vi "Initialise Indegrees1.vi"(8 "error in (no error)":errorcluster, 11 "Topological Sort in":refnum<class "Topological Sort.lvclass">) -> (0 "error out":errorcluster, 3 "Topological Sort out":refnum<class "Topological Sort.lvclass">)   [LabVIEW 2025, in "AOC.lvlib" / "Topological Sort.lvlib" / "Topological Sort.lvclass"]
uses:
  Topological Sort.lvclass
  Topological Sort.lvclass/Topological Sort.ctl
  Graph/Graph.lvclass
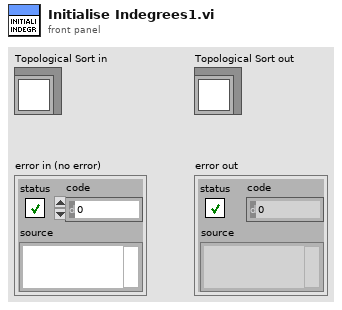
[diagram p1: front panel]
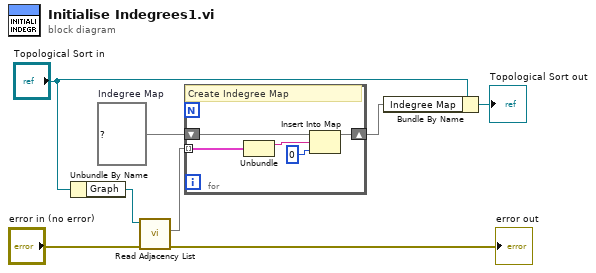
[diagram p0: block diagram]
diagram:
  w8 = map{string, u64} {}  # Indegree Map
  n1 = Unbundle By Name("Topological Sort in") -> ("Graph"=w7:refnum<class "Graph.lvclass">)
  n2 = call-dynamic "Read Adjacency List.vi"("error in (no error)"="error in (no error)", "Graph in"=w7) -> ("error out"=→"error out":errorcluster, "Adjacency List"=w6:map{string, string[]})  [unwired: 7 in, 1 out]
  n3 = for {
    shift-right: [w11] -> w4
    shift-left: w8 -> [w12]
    tunnel: w6 -> [w10] mode=indexing
    # "Create Indegree Map"
    n4 = Unbundle(w10) -> (w9:string)  [unwired: 1 out]
    n5 = Insert Into Map(map in=w12, key=w9, value=u64 0) -> (map out=w11:map{string, u64})  [unwired: 2 out]
  }
  n6 = Bundle By Name(cluster="Topological Sort in", "Indegree Map"=w4) -> (→"Topological Sort out":refnum<class "Topological Sort.lvclass">)
